vi "校正设置初始化.vi"() -> (3 "appended path":path)   [LabVIEW 2011]
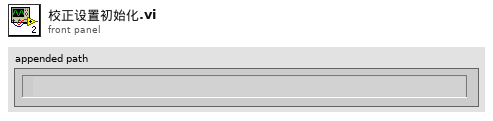
[diagram p1: front panel]
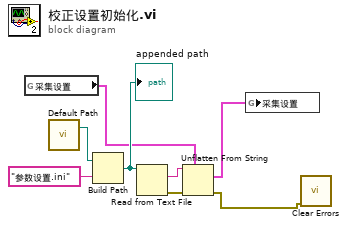
[diagram p0: block diagram]
diagram:
  n1 = global read "全局变量.vi" "采集设置"() -> (w3:cluster{"存储路径":path, "Device":u32, "采集间隔时间":u16})
  n2 = call "Default Path.vi"() -> ("Default Path data"=w4:path)  [unwired: 3 in, 1 out]
  n3 = Build Path(base path=w4, name or relative path="参数设置.ini" ("名称或相对路径")) -> (appended path=w6:path)
  "appended path" <- w6
  n4 = Read from Text File(file (use dialog)=w6) -> (text=w7:string, error out=w8:errorcluster)  [unwired: 3 in, 2 out]
  n5 = Unflatten From String(type=w3, binary string=w7, error in (no error)=w8) -> (value=w2:cluster{"存储路径":path, "Device":u32, "采集间隔时间":u16}, error out=w1:errorcluster)  [unwired: 2 in, 1 out]
  n6 = global write "全局变量.vi" "采集设置"(w2) -> ()
  n7 = call <vilib>:"Clear Errors.vi"("error in (no error)"=w1) -> ()  [unwired: 5 in, 2 out]
